vi "OPEN AND CONFIGURE.vi"(8 "error in SERIAL OPEN":errorcluster, 9 "array configuration":bool[](array[boolean]), 11 "VISA resource name":refnum<visa-resource-name>="COM3") -> (0 "error out SERIAL OPEN":errorcluster, 1 "configuration answer":string, 3 "VISA resource name out":refnum<visa-resource-name>)   [LabVIEW 2018]
uses:
  <vilib>/Instr/_visa.llb/VISA Configure Serial Port (Instr).vi
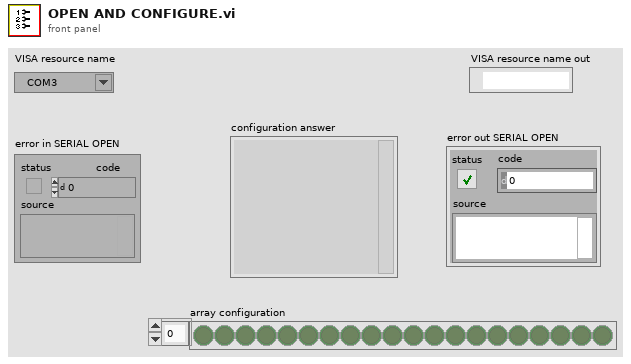
[diagram p1: front panel]
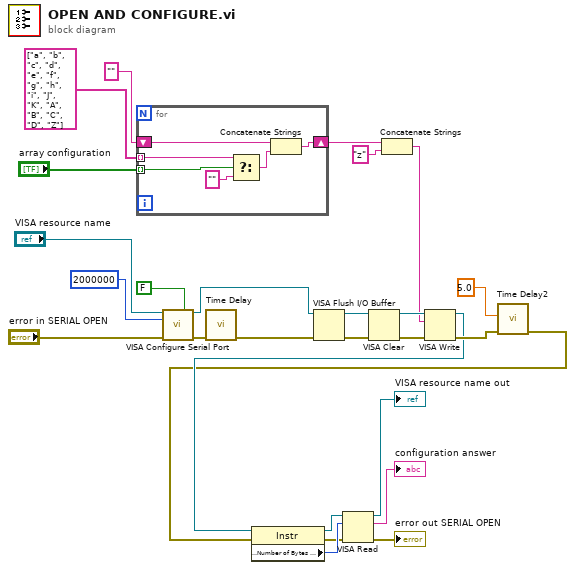
[diagram p0: block diagram]
diagram:
  n1 = for {
    tunnel: "array configuration" -> [w33] mode=indexing
    tunnel: string[] ["a", "b", "c", "d", "e", "f", "g", "h", "i", "J", "K", "A", "B", "C", "D", "Z"] ("Array") -> [w32] mode=indexing
    shift-right: [w28] -> w4
    shift-left: "" ("f") -> [w30]
    n2 = Select(t=w32, s=w33, f="") -> (s? t:f=w29:string)
    n3 = Concatenate Strings(w30, w29) -> (w28:string)
  }
  n4 = call-poly "VISA Configure Serial Port"("VISA resource name"="VISA resource name", "Enable Termination\nChar (T)"=FALSE ("Enable Termination\nChar (T)"), "baud rate (9600)"=u32 2000000, "error in (no error)"="error in SERIAL OPEN") -> ("VISA resource name out"=w24:refnum<visa-resource-name>, "error out"=w25:errorcluster)  [unwired: 10 in]
  n5 = call "Time Delay"("error in (no error)"=w25) -> ("error out"=w23:errorcluster)  [unwired: 10 in]
  n6 = VISA Flush I/O Buffer(VISA resource name=w24, error in (no error)=w23) -> (VISA resource name out=w22:refnum<visa-resource-name>, error out=w21:errorcluster)  [unwired: 1 in]
  n7 = VISA Clear(VISA resource name=w22, error in (no error)=w21) -> (VISA resource name out=w19:refnum<visa-resource-name>, error out=w20:errorcluster)
  n8 = Concatenate Strings(w4, "z" ("string")) -> (w2:string)
  n9 = VISA Write(VISA resource name=w19, write buffer=w2, error in (no error)=w20) -> (VISA resource name out=w14:refnum<visa-resource-name>, error out=w18:errorcluster)  [unwired: 1 out]
  n10 = call "Time Delay2"("error in (no error)"=w18, "Delay Time (s)"=5.0) -> ("error out"=w11:errorcluster)  [unwired: 9 in]
  n11 = property class="Instr"(reference=w14, error in=w11) -> (reference out=w15:refnum<visa-resource-name>, error out=w10:errorcluster, "Serial Settings:Number of Bytes at Serial Port"=w16:u32)
  n12 = VISA Read(VISA resource name=w15, byte count=w16, error in (no error)=w10) -> (VISA resource name out=→"VISA resource name out":refnum<visa-resource-name>, read buffer=→"configuration answer":string, error out=→"error out SERIAL OPEN":errorcluster)  [unwired: 1 out]
